vi "Tektronix TTR500 Series Application.vi"() -> ()   [LabVIEW 2012]
doc: "This VI illustrates typical measuring task for a network analyzer. It measures a band-pass filter (center frequency: 947.5 MHz), and calculates and displays its bandwidth, insertion loss, and so on.\n\nNote:\n(1) For this function you must set DUT on instrument."
uses:
  <instrlib>/Tektronix TTR500 Series/Tektronix TTR500 Series.lvlib
panel:
  in  "Save State (F: Disable)":bool
  in  "Reset? (T: Yes)":bool=TRUE
  in  "ID Query? (T: Yes)":bool=TRUE
  out "High":dbl
  out "Low":dbl
  out "Center Frequency":dbl format="%^.2e"
  out "Q Value":dbl format="%^.2e"
  out "Loss":dbl format="%^.2e"
  out "Bandwidth":dbl format="%^.2e"
  in  "VISA resource name":refnum<visa-resource-name>
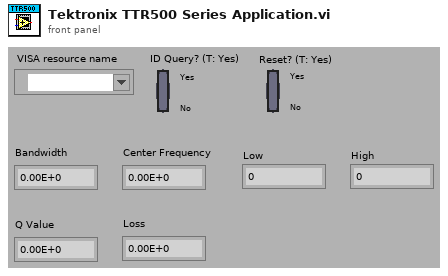
[diagram p1: front panel]
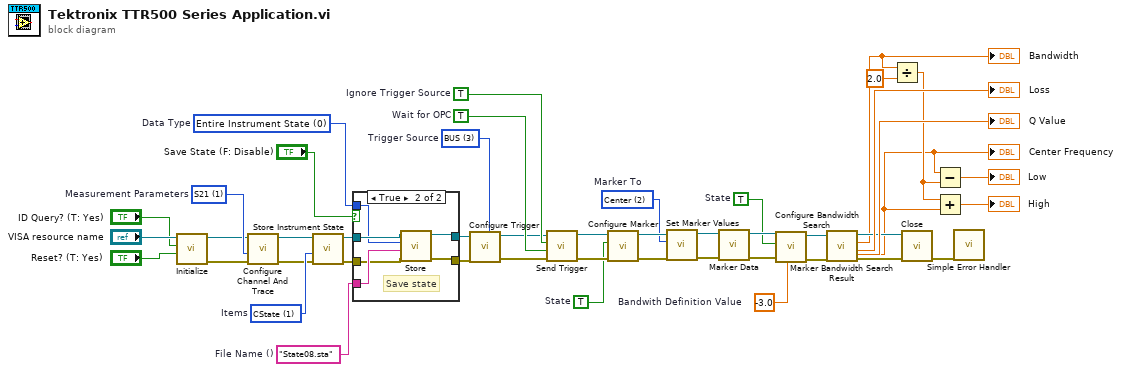
[diagram p0: block diagram]
diagram:
  w5 = u16 1 items=["S11", "S21", "S31", "S41", "S12", "S22", "S32", "S42", "S13", "S23", "S33", "S43", "S14", "S24", "S34", "S44", "A", "B", "C", "D", "R1", "R2", "R3", "R4"]  # Measurement Parameters
  w32 = -3.0  # Bandwith Definition Value
  w33 = TRUE  # State
  w38 = u16 2 items=["Start", "Stop", "Center", "Reference", "Electrical Delay"]  # Marker To
  w41 = TRUE  # State
  w44 = TRUE  # Wait for OPC
  w45 = TRUE  # Ignore Trigger Source
  w46 = u16 3 items=["Internal", "External", "Manual", "BUS"]  # Trigger Source
  w16 = "State08.sta"  # File Name ()
  w17 = u16 0 items=["Entire Instrument State", "Formatted Data Array", "Image On The LCD Display", "Segment Sweep Table", "Limit Table", "Power Sensor A", "Power Sensor B", "VBA Project", "Loss Compensation Table 1", "Loss Compensation Table 2", "Loss Compensation Table 3", "Loss Compensation Table 4"]  # Data Type
  w6 = u16 1 items=["State", "CState", "Dstate", "CDState"]  # Items
  n1 = call <instrlib>:"Initialize.vi"("Reset? (T: Yes)"="Reset? (T: Yes)", "ID Query? (T: Yes)"="ID Query? (T: Yes)", "VISA resource name"="VISA resource name") -> ("error out"=w3:errorcluster, "VISA resource name out"=w4:refnum<visa-resource-name>)  [unwired: 6 in, 1 out]
  n2 = call <instrlib>:"Configure Channel And Trace.vi"("error in (no error)"=w3, "Measurement Parameters (0: S11)"=w5, "VISA resource name"=w4) -> ("error out"=w1:errorcluster, "VISA resource name out"=w2:refnum<visa-resource-name>)  [unwired: 7 in]
  n3 = call <instrlib>:"Store Instrument State.vi"("error in (no error)"=w1, "Items (1: CState)"=w6, "VISA resource name"=w2) -> ("error out"=w7:errorcluster, "VISA resource name out"=w8:refnum<visa-resource-name>)  [unwired: 7 in]
  n4 = case shown="True" "Save State (F: Disable)" {
    tunnel: w17 -> [_ w51]
    tunnel: w16 -> [_ w50]
    tunnel: w8 -> [w48 w52]
    tunnel: [w48 w53] -> w15
    tunnel: w7 -> [w47 w49]
    tunnel: [w47 w54] -> w14
    frame False {
      # "Don't save"
    }
    frame True {
      # "Save state"
      n5 = call <instrlib>:"Store.vi"("error in (no error)"=w49, "File Name ()"=w50, "Data Type (0: Entire Instrument State)"=w51, "VISA resource name"=w52) -> ("error out"=w54:errorcluster, "VISA resource name out"=w53:refnum<visa-resource-name>)  [unwired: 6 in]
    }
  }
  n6 = call <instrlib>:"Configure Trigger.vi"("Trigger Source (0: Internal)"=w46, "error in (no error)"=w14, "VISA resource name"=w15) -> ("error out"=w9:errorcluster, "VISA resource name out"=w10:refnum<visa-resource-name>)  [unwired: 7 in]
  n7 = call <instrlib>:"Send Trigger.vi"("error in (no error)"=w9, "Wait for OPC (F: Do not Wait)"=w44, "Ignore Trigger Source (F: Do not Ignore)"=w45, "VISA resource name"=w10) -> ("error out"=w42:errorcluster, "VISA resource name out"=w43:refnum<visa-resource-name>)  [unwired: 6 in]
  n8 = call <instrlib>:"Configure Marker.vi"("error in (no error)"=w42, "Marker State (F: Disabled)"=w41, "VISA resource name"=w43) -> ("error out"=w39:errorcluster, "VISA resource name out"=w40:refnum<visa-resource-name>)  [unwired: 7 in]
  n9 = call <instrlib>:"Set Marker Values.vi"("error in (no error)"=w39, "Marker To (0: Start)"=w38, "VISA resource name"=w40) -> ("error out"=w36:errorcluster, "VISA resource name out"=w37:refnum<visa-resource-name>)  [unwired: 7 in]
  n10 = call <instrlib>:"Marker Data.vi"("error in (no error)"=w36, "VISA resource name"=w37) -> ("error out"=w34:errorcluster, "VISA resource name out"=w35:refnum<visa-resource-name>)  [unwired: 5 in, 3 out]
  n11 = call <instrlib>:"Configure Bandwidth Search.vi"("Bandwidth Definition Value (-3.0)"=w32, "error in (no error)"=w34, "Result Display State (F: Disable)"=w33, "VISA resource name"=w35) -> ("error out"=w30:errorcluster, "VISA resource name out"=w31:refnum<visa-resource-name>)  [unwired: 6 in]
  n12 = call <instrlib>:"Marker Bandwidth Search Result.vi"("error in (no error)"=w30, "VISA resource name"=w31) -> ("error out"=w26:errorcluster, "Loss"=→"Loss":dbl, "Bandwidth"=w25:dbl, "VISA resource name out"=w27:refnum<visa-resource-name>, "Q Value"=→"Q Value":dbl, "Center Frequency"=w21:dbl)  [unwired: 4 in]
  "Bandwidth" <- w25
  "Center Frequency" <- w21
  n13 = Divide(x=w25, y=2.0) -> (x/y=w22:dbl)
  n14 = call <instrlib>:"Close.vi"("error in (no error)"=w26, "VISA resource name"=w27) -> ("error out"=w19:errorcluster)  [unwired: 9 in]
  n15 = Subtract(x=w21, y=w22) -> (x-y=→"Low":dbl)
  n16 = Add(x=w22, y=w21) -> (x+y=→"High":dbl)
  n17 = call <vilib>:"Simple Error Handler.vi"("error in (no error)"=w19) -> ()  [unwired: 4 in, 5 out]
